vi "ACQ enkoders reset.vi"(6 "Reset":bool, 8 "error in (no error)":errorcluster, 11 "Tasks ref in":T1) -> (0 "error out":errorcluster, 3 "Tasks ref out":T1)   [LabVIEW 2014]
doc: "Use this template to build a VI to use as a subVI."
uses:
  Kontrolki/KartaDAQ/ACQ all read tasks.ctl
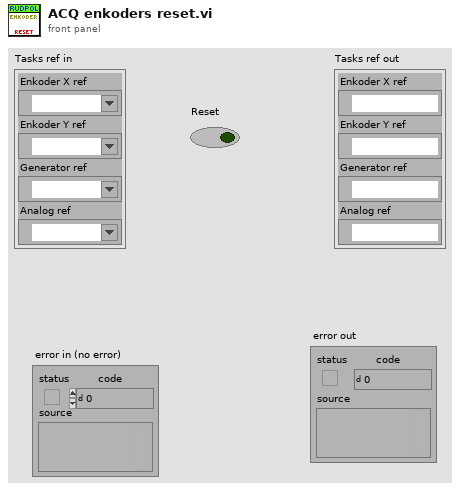
[diagram p1: front panel]
types:
  T1 = typedef "ACQ all read tasks.ctl" = cluster{"Enkoder X ref":refnum<k21>, "Enkoder Y ref":refnum<k21>, "Generator ref":refnum<k21>, "Analog ref":refnum<k21>}
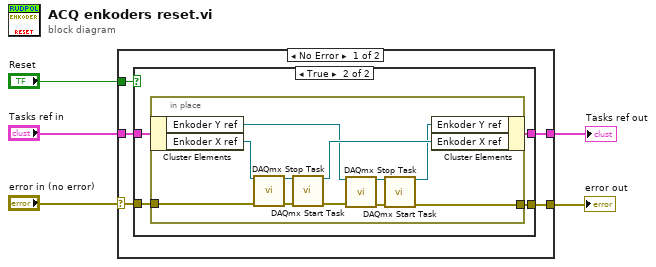
[diagram p0: block diagram]
diagram:
  n1 = case shown="No Error" "error in (no error)" {
    selector: "error in (no error)" -> [w10 w29]
    tunnel: [w8 w29] -> w4
    tunnel: "Tasks ref in" -> [w9 w28]
    tunnel: [w7 w28] -> w2
    tunnel: "Reset" -> [w6 _]
    frame No Error {
      n2 = case shown="True" w6 {
        tunnel: w10 -> [w11 w16]
        tunnel: w9 -> [w12 w15]
        tunnel: [w11 w14] -> w8
        tunnel: [w12 w13] -> w7
        frame False {
        }
        frame True {
          n3 = in-place {
            in-place-border: w16 -> [w25]
            in-place-border: [w17] -> w14
            n4 = in-place-cluster #1(w15) -> ("Enkoder Y ref"=w19:refnum<k21>, "Enkoder X ref"=w26:refnum<k21>)
            n5 = call <vilib>:"DAQmx Stop Task.vi"("task/channels in"=w26, "error in"=w25) -> ("task out"=w24:refnum<k21>, "error out"=w27:errorcluster)  [unwired: 12 in]
            n6 = call <vilib>:"DAQmx Start Task.vi"("task/channels in"=w24, "error in"=w27) -> ("task out"=w23:refnum<k21>, "error out"=w20:errorcluster)  [unwired: 12 in]
            n7 = call <vilib>:"DAQmx Stop Task.vi"("task/channels in"=w19, "error in"=w20) -> ("task out"=w22:refnum<k21>, "error out"=w21:errorcluster)  [unwired: 12 in]
            n8 = call <vilib>:"DAQmx Start Task.vi"("task/channels in"=w22, "error in"=w21) -> ("task out"=w18:refnum<k21>, "error out"=w17:errorcluster)  [unwired: 12 in]
            n9 = in-place-cluster #1("Enkoder Y ref"=w18, "Enkoder X ref"=w23) -> (w13:T1)
          }
        }
      }
    }
    frame Error {
    }
  }
  "error out" <- w4
  "Tasks ref out" <- w2
